vi "aquire_channels.vi"(0 "instrument handle":refnum<k15>, 2 "Controls Cluster":T5 {"C1 vertical coupling / V" items=["AC", "DC", "Ground"]; "C2 vertical coupling / V" items=["AC", "DC", "Ground"]; "Trigger slope" items=["Positive", "Negative"]}, 11 "error in":errorcluster, 12 "scope Q data in":T1) -> (4 "instrument handle out":refnum<k15>, 14 "scope Q data out":T1, 15 "error out":errorcluster)   [LabVIEW 2023]
uses:
  <instrlib>/niScope/Controls/niScope vertical coupling.ctl
  <instrlib>/niScope/Controls/niScope trigger source.ctl
  <instrlib>/niScope/Controls/niScope trigger slope.ctl
  <instrlib>/niScope/Acquire/Fetch/niScope Fetch WDT.vi
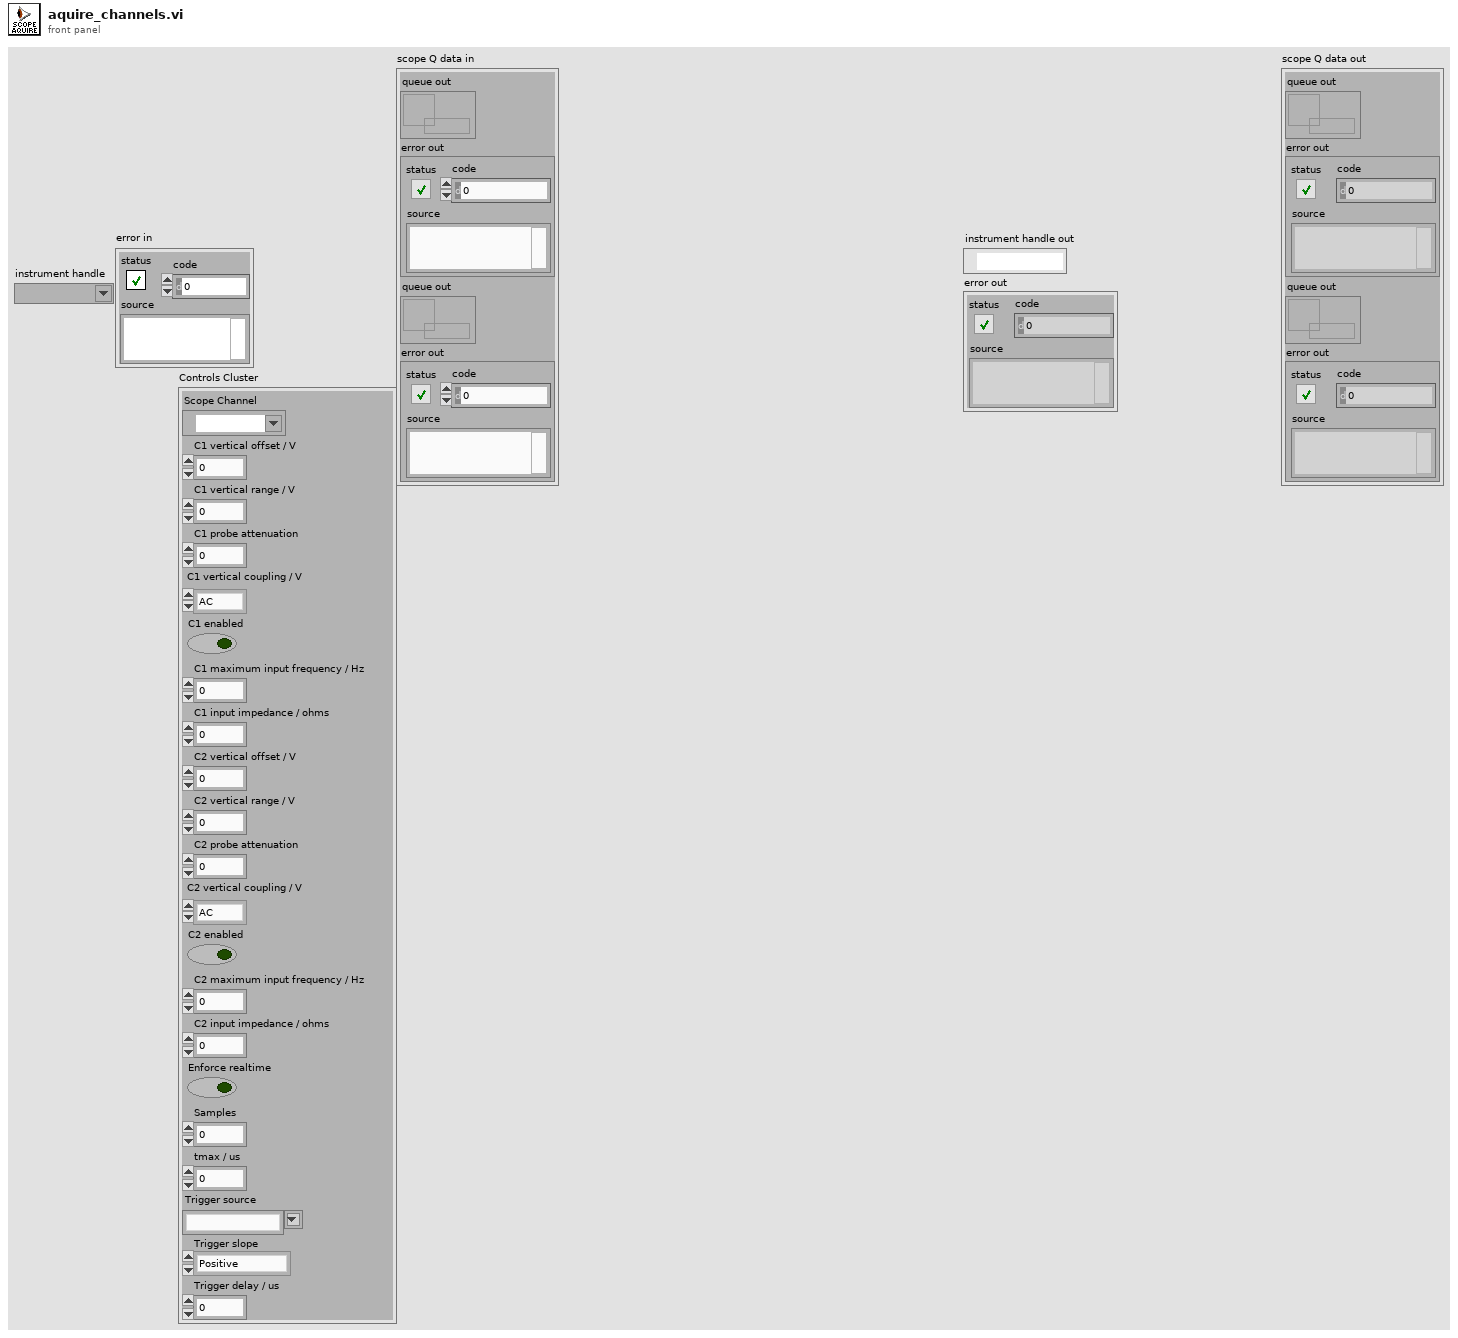
[diagram p1: front panel]
types:
  T1 = cluster{"queue out":refnum<queue>, "error out":errorcluster, "queue out":refnum<queue>, "error out":errorcluster}
  T2 = typedef "niScope vertical coupling.ctl" = i32
  T3 = typedef "niScope trigger source.ctl" = string
  T4 = typedef "niScope trigger slope.ctl" = i32
  T5 = cluster{"Scope Channel":refnum<k15>, "C1 vertical offset / V":dbl, "C1 vertical range / V":dbl, "C1 probe attenuation":dbl, "C1 vertical coupling / V":T2, "C1 enabled":bool, "C1 maximum input frequency / Hz":dbl, "C1 input impedance / ohms":u32, "C2 vertical offset / V":dbl, "C2 vertical range / V":dbl, "C2 probe attenuation":dbl, "C2 vertical coupling / V":T2, "C2 enabled":bool, "C2 maximum input frequency / Hz":dbl, "C2 input impedance / ohms":u32, "Enforce realtime":bool, "Samples":i64, "tmax / us ":dbl, "Trigger source":T3, "Trigger slope":T4, "Trigger delay / us":dbl}
  T6 = cluster{"actualSamples":i32, "absoluteInitialX":dbl, "relativeInitialX":dbl, "xIncrement":dbl, "offset":dbl, "gain":dbl, "reserved1":dbl, "reserved2":dbl}
  T7 = cluster{"wfm info":cluster{"actualSamples":i32, "absoluteInitialX":dbl, "relativeInitialX":dbl, "xIncrement":dbl, "offset":dbl, "gain":dbl, "reserved1":dbl, "reserved2":dbl}, "wfm":waveform(dbl), bool}
  T8 = cluster{"wfm info":cluster{"actualSamples":i32, "absoluteInitialX":dbl, "relativeInitialX":dbl, "xIncrement":dbl, "offset":dbl, "gain":dbl, "reserved1":dbl, "reserved2":dbl}, "Offset WFm":waveform(dbl), bool}
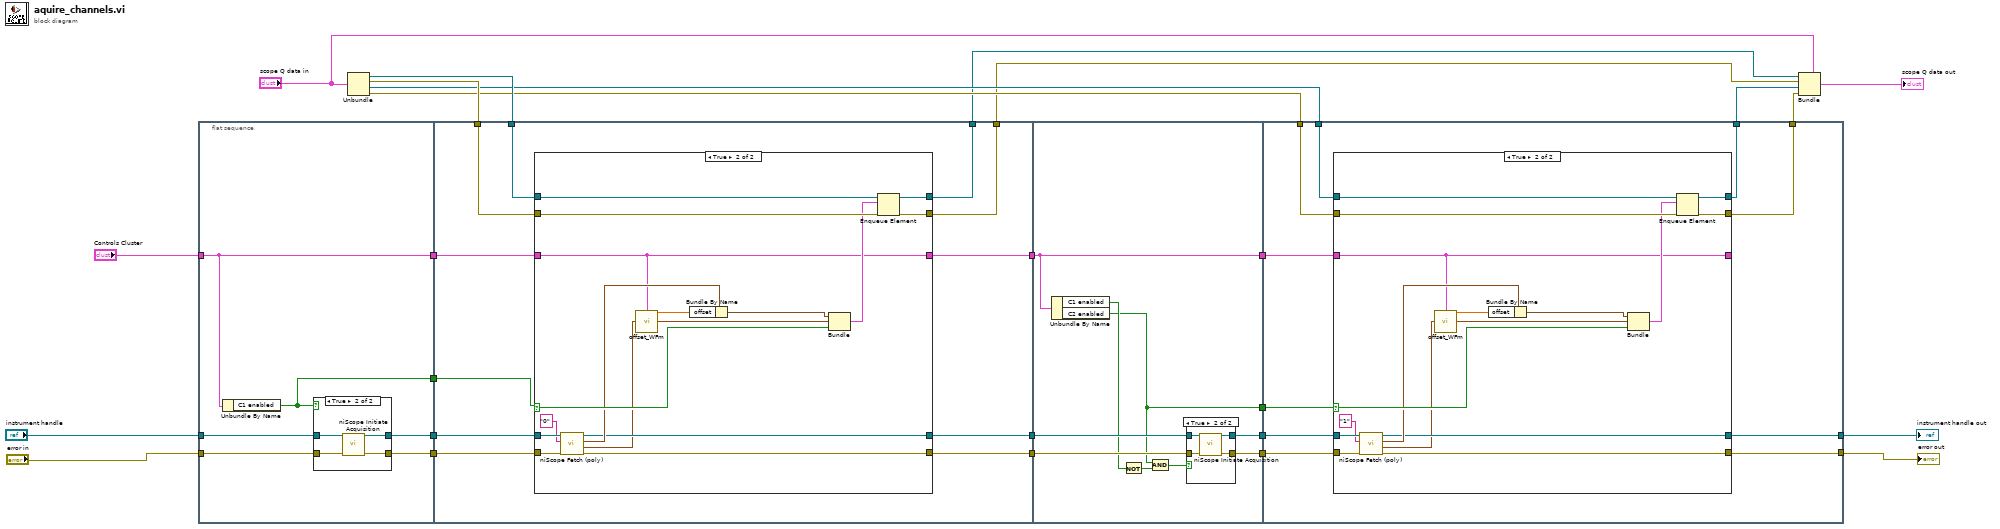
[diagram p0: block diagram]
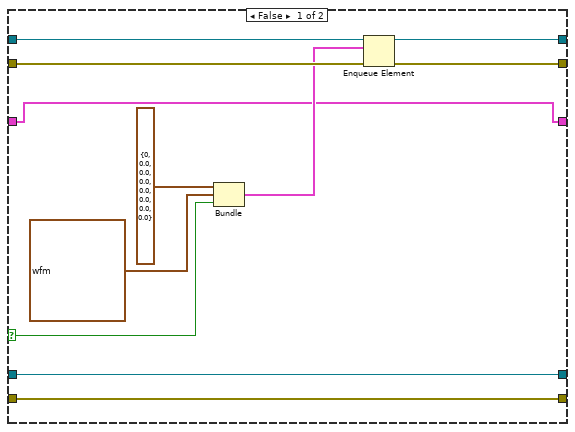
[diagram p3: hidden frame]
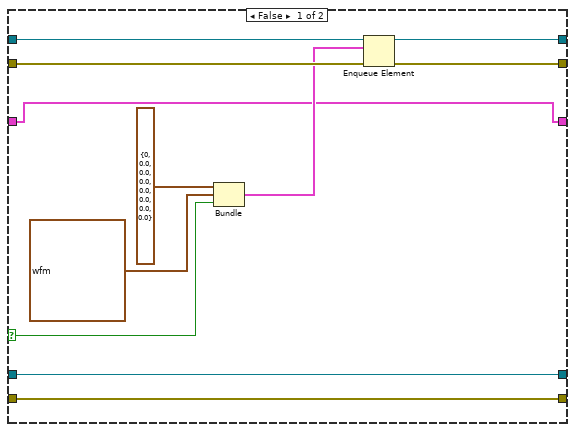
[diagram p5: hidden frame]
diagram:
  n1 = flat-sequence {
    tunnel: [w32] -> w24
    tunnel: [w31] -> w23
    tunnel: "instrument handle" -> [w30]
    tunnel: "error in" -> [w29]
    tunnel: "Controls Cluster" -> [w28]
    tunnel: [w28] -> w17
    tunnel: [w27] -> w15
    tunnel: w25 -> [w49]
    tunnel: w26 -> [w48]
    tunnel: w24 -> [w47]
    tunnel: w23 -> [w46]
    tunnel: [w45] -> w7
    tunnel: [w44] -> w6
    tunnel: [w43] -> w20
    tunnel: [w42] -> w19
    tunnel: w17 -> [w41]
    tunnel: [w40] -> w16
    tunnel: w15 -> [w39]
    tunnel: w20 -> [w84]
    tunnel: w19 -> [w83]
    tunnel: w16 -> [w81]
    tunnel: [w81] -> w14
    tunnel: [w80] -> w13
    tunnel: [w79] -> w12
    tunnel: [w78] -> w11
    tunnel: w14 -> [w102]
    tunnel: w13 -> [w100]
    tunnel: w12 -> [w99]
    tunnel: w11 -> [w101]
    tunnel: w10 -> [w98]
    tunnel: w9 -> [w97]
    tunnel: [w96] -> w5
    tunnel: [w95] -> w4
    tunnel: [w94] -> w2
    tunnel: [w93] -> w1
    frame #0 {
      n2 = Unbundle By Name(w28) -> ("C1 enabled"=w27:bool)
      n3 = case shown="True" w27 {
        tunnel: [w34 w38] -> w32
        tunnel: [w33 w37] -> w31
        tunnel: w30 -> [w34 w36]
        tunnel: w29 -> [w33 w35]
        frame False {
        }
        frame True {
          n4 = call <instrlib>:"niScope Initiate Acquisition.vi"("instrument handle"=w36, "error in"=w35) -> ("instrument handle out"=w38:refnum<k15>, "error out"=w37:errorcluster)  [unwired: 12 in]
        }
      }
    }
    frame #1 {
      n5 = case shown="True" w39 {
        selector: w39 -> [w58 w77]
        tunnel: w49 -> [w57 w76]
        tunnel: w48 -> [w56 w75]
        tunnel: [w55 w74] -> w45
        tunnel: [w54 w73] -> w44
        tunnel: [w51 w67] -> w43
        tunnel: [w50 w66] -> w42
        tunnel: w47 -> [w51 w65]
        tunnel: w46 -> [w50 w64]
        tunnel: [w52 w62] -> w40
        tunnel: w41 -> [w52 w62]
        frame False {
          n6 = Bundle("wfm info"=T6 {"actualSamples"=0, "absoluteInitialX"=0.0, "relativeInitialX"=0.0, "xIncrement"=0.0, "offset"=0.0, "gain"=0.0, "reserved1"=0.0, "reserved2"=0.0}, "wfm"=waveform(dbl) {"t0"=timestamp(0 s since 1904-01-01), "dt"=0.0, "Y"=[]}, w58) -> (w53:T7)  [unwired: 1 in]
          n7 = Enqueue Element(queue=w57, element=w53, error in (no error)=w56) -> (queue out=w55:refnum<queue>, error out=w54:errorcluster)  [unwired: 1 in, 1 out]
        }
        frame True {
          n8 = call-poly <instrlib>:"niScope Fetch (poly).vi"("error in"=w64, "channels"="0", "instrument handle"=w65) -> ("error out"=w66:errorcluster, "wfm"=w63:waveform(dbl), "wfm info"=w69:T6, "instrument handle out"=w67:refnum<k15>)  [unwired: 5 in]
          n9 = call "offset_WFm.vi"("Controls Cluster"=w62, "WFm"=w63) -> ("WFm Offset / s"=w70:dbl, "Offset WFm"=w71:waveform(dbl))  [unwired: 12 in]
          n10 = Bundle By Name(cluster=w69, "offset"=w70) -> (w68:T6)
          n11 = Bundle("wfm info"=w68, "Offset WFm"=w71, w77) -> (w72:T8)  [unwired: 1 in]
          n12 = Enqueue Element(queue=w76, element=w72, error in (no error)=w75) -> (queue out=w74:refnum<queue>, error out=w73:errorcluster)  [unwired: 1 in, 1 out]
        }
      }
    }
    frame #2 {
      n13 = Unbundle By Name(w81) -> ("C1 enabled"=w82:bool, "C2 enabled"=w78:bool)
      n14 = Not(x=w82) -> (.not. x?=w86:bool)
      n15 = And(x=w78, y=w86) -> (x .and. y?=w85:bool)
      n16 = case shown="True" w85 {
        tunnel: w84 -> [w88 w92]
        tunnel: w83 -> [w87 w91]
        tunnel: [w88 w90] -> w80
        tunnel: [w87 w89] -> w79
        frame False {
        }
        frame True {
          n17 = call <instrlib>:"niScope Initiate Acquisition.vi"("instrument handle"=w92, "error in"=w91) -> ("instrument handle out"=w90:refnum<k15>, "error out"=w89:errorcluster)  [unwired: 12 in]
        }
      }
    }
    frame #3 {
      n18 = case shown="True" w101 {
        selector: w101 -> [w111 w130]
        tunnel: w98 -> [w110 w129]
        tunnel: w97 -> [w109 w128]
        tunnel: [w108 w127] -> w96
        tunnel: [w107 w126] -> w95
        tunnel: [w104 w120] -> w94
        tunnel: [w103 w119] -> w93
        tunnel: w100 -> [w104 w118]
        tunnel: w99 -> [w103 w117]
        tunnel: [w105 w115] -> _
        tunnel: w102 -> [w105 w115]
        frame False {
          n19 = Bundle("wfm info"=T6 {"actualSamples"=0, "absoluteInitialX"=0.0, "relativeInitialX"=0.0, "xIncrement"=0.0, "offset"=0.0, "gain"=0.0, "reserved1"=0.0, "reserved2"=0.0}, "wfm"=waveform(dbl) {"t0"=timestamp(0 s since 1904-01-01), "dt"=0.0, "Y"=[]}, w111) -> (w106:T7)  [unwired: 1 in]
          n20 = Enqueue Element(queue=w110, element=w106, error in (no error)=w109) -> (queue out=w108:refnum<queue>, error out=w107:errorcluster)  [unwired: 1 in, 1 out]
        }
        frame True {
          n21 = call-poly <instrlib>:"niScope Fetch (poly).vi"("error in"=w117, "channels"="1", "instrument handle"=w118) -> ("error out"=w119:errorcluster, "wfm"=w116:waveform(dbl), "wfm info"=w122:T6, "instrument handle out"=w120:refnum<k15>)  [unwired: 5 in]
          n22 = call "offset_WFm.vi"("Controls Cluster"=w115, "WFm"=w116) -> ("WFm Offset / s"=w123:dbl, "Offset WFm"=w124:waveform(dbl))  [unwired: 12 in]
          n23 = Bundle By Name(cluster=w122, "offset"=w123) -> (w121:T6)
          n24 = Bundle("wfm info"=w121, "Offset WFm"=w124, w130) -> (w125:T8)  [unwired: 1 in]
          n25 = Enqueue Element(queue=w129, element=w125, error in (no error)=w128) -> (queue out=w127:refnum<queue>, error out=w126:errorcluster)  [unwired: 1 in, 1 out]
        }
      }
    }
  }
  n26 = Unbundle("scope Q data in") -> ("queue out"=w25:refnum<queue>, "error out"=w26:errorcluster, "queue out"=w10:refnum<queue>, "error out"=w9:errorcluster)
  n27 = Bundle(cluster="scope Q data in", "queue out"=w7, "error out"=w6, "queue out"=w5, "error out"=w4) -> (→"scope Q data out":T1)
  "instrument handle out" <- w2
  "error out" <- w1
